vi "Finish.vi"   [LabVIEW 2020]
doc: "This VIcloses device references, sends final commands to the network tables and the joysticks, and terminates all command and control loops."
uses:
  GlobalDrivebase.vi
  GlobalDriverStationCommands.vi
  <vilib>/Rock Robotics/WPI/Utilities/WPI_GetSetVariantRefNum.vi
  GlobalMiscellaneous.vi
  GlobalActuators.vi
types:
  T1 = typedef "WPI_JoystickDevRef.ctl" = cluster{"Device":T2}
  T2 = typedef "WPI_JoystickDeviceEnum.ctl" = enum16{"USB 0", "USB 1", "USB 2", "USB 3", "USB 4", "USB 5"}
  T3 = typedef "WPI_PWMDeviceRef.ctl" = cluster{"DeviceStatus":errorcluster, "PWM Channel":T4}
  T4 = typedef "FPGA_DIOPWMChannel.ctl" = enum8{"PWM 0", "PWM 1", "PWM 2", "PWM 3", "PWM 4", "PWM 5", "PWM 6", "PWM 7", "PWM 8", "PWM 9", "PWM MXP 0", "PWM MXP 1", "PWM MXP 2", "PWM MXP 3", "PWM MXP 4", "PWM MXP 5", "PWM MXP 6", "PWM MXP 7", "PWM MXP 8", "PWM MXP 9", "Invalid"}
  T5 = typedef "WPI_MotorControlDeviceRef.ctl" = cluster{"DeviceStatus":errorcluster, "Type":T6, "PWM":cluster{"PWM Channel":T4, "DeadBand":T7}, "CAN":cluster{"Device Number":u8, "SetOutput VI Ref":variant, "GetOutput VI Ref":variant, "Enable VI Ref":variant, "Disable VI Ref":variant, "Data":variant}, "Invert":bool, "DIO PWM":cluster{"PWM \"Enable\" Channel":T4, "DIOChannel":T8, "PWM Rate":dbl}}
  T6 = typedef "WPI_MotorControlType.ctl" = enum16{"PWM", "CAN", "DIO PWM"}
  T7 = typedef "WPI_PWMDeadband.ctl" = cluster{"Name":string, "maxPositivePwm":i32, "minPositivePwm":i32, "centerPwm":i32, "maxNegativePwm":i32, "minNegativePwm":i32, "angularRange":u16}
  T8 = typedef "FPGA_DIOChannel.ctl" = enum8{"DIO 0", "DIO 1", "DIO 2", "DIO 3", "DIO 4", "DIO 5", "DIO 6", "DIO 7", "DIO 8", "DIO 9", "DIO MXP 0", "DIO MXP 1", "DIO MXP 2", "DIO MXP 3", "DIO MXP 4", "DIO MXP 5", "DIO MXP 6", "DIO MXP 7", "DIO MXP 8", "DIO MXP 9", "DIO MXP 10", "DIO MXP 11", "DIO MXP 12", "DIO MXP 13", "DIO MXP 14", "DIO MXP 15", "SPI Port CS1", "SPI Port CS2", "SPI Port CS3", "SPI Port MISO", "SPI Port MOSI", "Invalid"}
  T9 = typedef "WPI_SolenoidDevRef.ctl" = cluster{"DevStatus":errorcluster, "Pneumatics Control Module":u8, "Forward Solenoid Channel":T10, "Reverse Solenoid Channel":T10}
  T10 = typedef "WPI_SolenoidChannel.ctl" = enum8{"Solenoid 0", "Solenoid 1", "Solenoid 2", "Solenoid 3", "Solenoid 4", "Solenoid 5", "Solenoid 6", "Solenoid 7", "Solenoid 8", "Solenoid 9", "Solenoid 10", "Solenoid 11", "Solenoid 12", "Solenoid 13", "Solenoid 14", "Solenoid 15", "Invalid"}
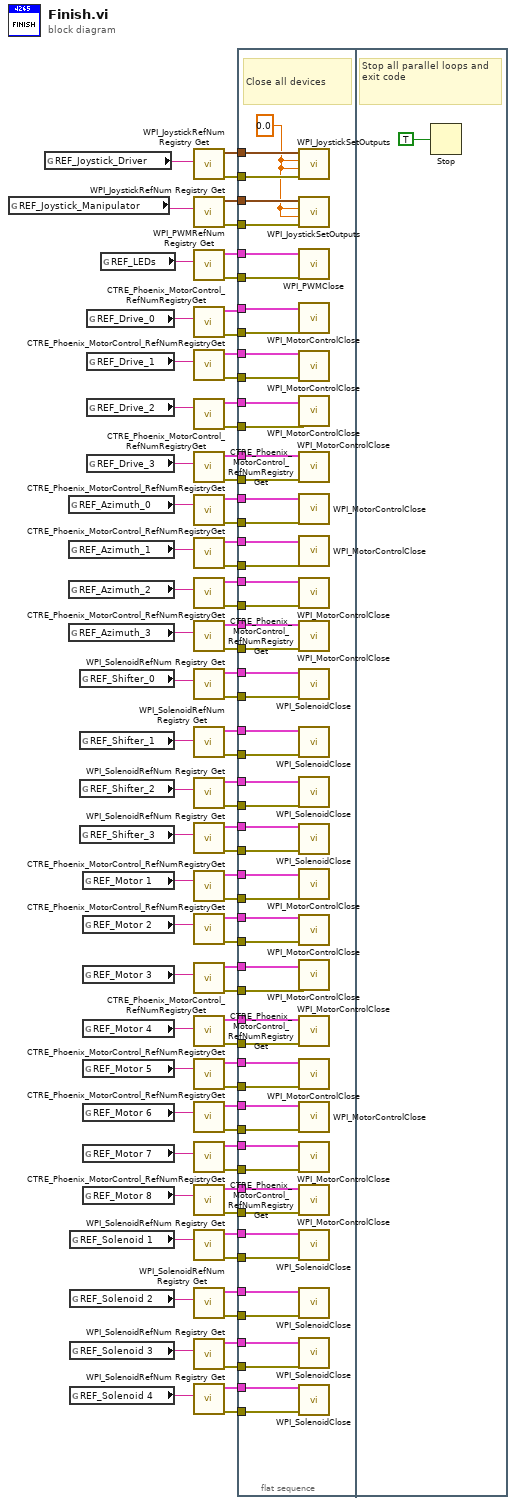
[diagram p0: block diagram]
diagram:
  n1 = global read "GlobalDriverStationCommands.vi" "REF_Joystick_Manipulator"() -> (w40:string)
  n2 = global read "GlobalDriverStationCommands.vi" "REF_Joystick_Driver"() -> (w41:string)
  n3 = global read "GlobalDrivebase.vi" "REF_Azimuth_0"() -> (w53:string)
  n4 = global read "GlobalDrivebase.vi" "REF_Azimuth_1"() -> (w52:string)
  n5 = global read "GlobalDrivebase.vi" "REF_Azimuth_2"() -> (w51:string)
  n6 = global read "GlobalDrivebase.vi" "REF_Azimuth_3"() -> (w50:string)
  n7 = global read "GlobalActuators.vi" "REF_Solenoid 1"() -> (w9:string)
  n8 = global read "GlobalActuators.vi" "REF_Solenoid 2"() -> (w10:string)
  n9 = global read "GlobalActuators.vi" "REF_Solenoid 3"() -> (w11:string)
  n10 = global read "GlobalActuators.vi" "REF_Solenoid 4"() -> (w12:string)
  n11 = global read "GlobalDrivebase.vi" "REF_Shifter_0"() -> (w45:string)
  n12 = global read "GlobalDrivebase.vi" "REF_Shifter_1"() -> (w44:string)
  n13 = global read "GlobalDrivebase.vi" "REF_Shifter_2"() -> (w43:string)
  n14 = global read "GlobalDrivebase.vi" "REF_Shifter_3"() -> (w42:string)
  n15 = global read "GlobalActuators.vi" "REF_Motor 1"() -> (w1:string)
  n16 = global read "GlobalActuators.vi" "REF_Motor 2"() -> (w2:string)
  n17 = global read "GlobalActuators.vi" "REF_Motor 3"() -> (w3:string)
  n18 = global read "GlobalActuators.vi" "REF_Motor 4"() -> (w4:string)
  n19 = global read "GlobalActuators.vi" "REF_Motor 5"() -> (w5:string)
  n20 = global read "GlobalActuators.vi" "REF_Motor 6"() -> (w6:string)
  n21 = global read "GlobalActuators.vi" "REF_Motor 7"() -> (w7:string)
  n22 = global read "GlobalActuators.vi" "REF_Motor 8"() -> (w8:string)
  n23 = global read "GlobalDrivebase.vi" "REF_Drive_0"() -> (w49:string)
  n24 = global read "GlobalDrivebase.vi" "REF_Drive_1"() -> (w48:string)
  n25 = global read "GlobalDrivebase.vi" "REF_Drive_2"() -> (w47:string)
  n26 = global read "GlobalDrivebase.vi" "REF_Drive_3"() -> (w46:string)
  n27 = global read "GlobalMiscellaneous.vi" "REF_LEDs"() -> (w37:string)
  n28 = call <vilib>:"WPI_JoystickRefNum Registry Get.vi"("refnum name"=w41) -> ("error out"=w80:errorcluster, "JoystickDevRef"=w81:T1)  [unwired: 9 in]
  n29 = call <vilib>:"WPI_JoystickRefNum Registry Get.vi"("refnum name"=w40) -> ("error out"=w78:errorcluster, "JoystickDevRef"=w79:T1)  [unwired: 9 in]
  n30 = call <vilib>:"WPI_PWMRefNum Registry Get.vi"("refnum name"=w37) -> ("error out"=w38:errorcluster, "PWMDeviceRef"=w39:T3)  [unwired: 9 in]
  n31 = call <vilib>:"CTRE_Phoenix_MotorControl_RefNumRegistryGet.vi"("refnum name"=w49) -> ("error out"=w72:errorcluster, "PhoenixMotorControlDevRef"=w73:T5)  [unwired: 9 in]
  n32 = call <vilib>:"CTRE_Phoenix_MotorControl_RefNumRegistryGet.vi"("refnum name"=w48) -> ("error out"=w68:errorcluster, "PhoenixMotorControlDevRef"=w71:T5)  [unwired: 9 in]
  n33 = call <vilib>:"CTRE_Phoenix_MotorControl_RefNumRegistryGet.vi"("refnum name"=w47) -> ("error out"=w69:errorcluster, "PhoenixMotorControlDevRef"=w70:T5)  [unwired: 9 in]
  n34 = call <vilib>:"CTRE_Phoenix_MotorControl_RefNumRegistryGet.vi"("refnum name"=w46) -> ("error out"=w76:errorcluster, "PhoenixMotorControlDevRef"=w77:T5)  [unwired: 9 in]
  n35 = call <vilib>:"CTRE_Phoenix_MotorControl_RefNumRegistryGet.vi"("refnum name"=w53) -> ("error out"=w63:errorcluster, "PhoenixMotorControlDevRef"=w67:T5)  [unwired: 9 in]
  n36 = call <vilib>:"CTRE_Phoenix_MotorControl_RefNumRegistryGet.vi"("refnum name"=w52) -> ("error out"=w62:errorcluster, "PhoenixMotorControlDevRef"=w66:T5)  [unwired: 9 in]
  n37 = call <vilib>:"CTRE_Phoenix_MotorControl_RefNumRegistryGet.vi"("refnum name"=w51) -> ("error out"=w61:errorcluster, "PhoenixMotorControlDevRef"=w65:T5)  [unwired: 9 in]
  n38 = call <vilib>:"CTRE_Phoenix_MotorControl_RefNumRegistryGet.vi"("refnum name"=w50) -> ("error out"=w60:errorcluster, "PhoenixMotorControlDevRef"=w64:T5)  [unwired: 9 in]
  n39 = call <vilib>:"WPI_SolenoidRefNum Registry Get.vi"("refnum name"=w45) -> ("error out"=w58:errorcluster, "SolenoidDevRef"=w59:T9)  [unwired: 9 in]
  n40 = call <vilib>:"WPI_SolenoidRefNum Registry Get.vi"("refnum name"=w44) -> ("error out"=w56:errorcluster, "SolenoidDevRef"=w57:T9)  [unwired: 9 in]
  n41 = call <vilib>:"WPI_SolenoidRefNum Registry Get.vi"("refnum name"=w43) -> ("error out"=w54:errorcluster, "SolenoidDevRef"=w55:T9)  [unwired: 9 in]
  n42 = call <vilib>:"WPI_SolenoidRefNum Registry Get.vi"("refnum name"=w42) -> ("error out"=w74:errorcluster, "SolenoidDevRef"=w75:T9)  [unwired: 9 in]
  n43 = call <vilib>:"CTRE_Phoenix_MotorControl_RefNumRegistryGet.vi"("refnum name"=w1) -> ("error out"=w24:errorcluster, "PhoenixMotorControlDevRef"=w23:T5)  [unwired: 9 in]
  n44 = call <vilib>:"CTRE_Phoenix_MotorControl_RefNumRegistryGet.vi"("refnum name"=w2) -> ("error out"=w28:errorcluster, "PhoenixMotorControlDevRef"=w25:T5)  [unwired: 9 in]
  n45 = call <vilib>:"CTRE_Phoenix_MotorControl_RefNumRegistryGet.vi"("refnum name"=w3) -> ("error out"=w27:errorcluster, "PhoenixMotorControlDevRef"=w26:T5)  [unwired: 9 in]
  n46 = call <vilib>:"CTRE_Phoenix_MotorControl_RefNumRegistryGet.vi"("refnum name"=w4) -> ("error out"=w22:errorcluster, "PhoenixMotorControlDevRef"=w21:T5)  [unwired: 9 in]
  n47 = call <vilib>:"CTRE_Phoenix_MotorControl_RefNumRegistryGet.vi"("refnum name"=w5) -> ("error out"=w33:errorcluster, "PhoenixMotorControlDevRef"=w29:T5)  [unwired: 9 in]
  n48 = call <vilib>:"CTRE_Phoenix_MotorControl_RefNumRegistryGet.vi"("refnum name"=w6) -> ("error out"=w34:errorcluster, "PhoenixMotorControlDevRef"=w30:T5)  [unwired: 9 in]
  n49 = call <vilib>:"CTRE_Phoenix_MotorControl_RefNumRegistryGet.vi"("refnum name"=w7) -> ("error out"=w35:errorcluster, "PhoenixMotorControlDevRef"=w31:T5)  [unwired: 9 in]
  n50 = call <vilib>:"CTRE_Phoenix_MotorControl_RefNumRegistryGet.vi"("refnum name"=w8) -> ("error out"=w36:errorcluster, "PhoenixMotorControlDevRef"=w32:T5)  [unwired: 9 in]
  n51 = call <vilib>:"WPI_SolenoidRefNum Registry Get.vi"("refnum name"=w9) -> ("error out"=w16:errorcluster, "SolenoidDevRef"=w15:T9)  [unwired: 9 in]
  n52 = call <vilib>:"WPI_SolenoidRefNum Registry Get.vi"("refnum name"=w10) -> ("error out"=w18:errorcluster, "SolenoidDevRef"=w17:T9)  [unwired: 9 in]
  n53 = call <vilib>:"WPI_SolenoidRefNum Registry Get.vi"("refnum name"=w11) -> ("error out"=w20:errorcluster, "SolenoidDevRef"=w19:T9)  [unwired: 9 in]
  n54 = call <vilib>:"WPI_SolenoidRefNum Registry Get.vi"("refnum name"=w12) -> ("error out"=w14:errorcluster, "SolenoidDevRef"=w13:T9)  [unwired: 9 in]
  n55 = flat-sequence {
    tunnel: w73 -> [w136]
    tunnel: w71 -> [w135]
    tunnel: w72 -> [w134]
    tunnel: w81 -> [w133]
    tunnel: w80 -> [w132]
    tunnel: w79 -> [w131]
    tunnel: w78 -> [w130]
    tunnel: w77 -> [w128]
    tunnel: w76 -> [w127]
    tunnel: w75 -> [w126]
    tunnel: w74 -> [w125]
    tunnel: w70 -> [w124]
    tunnel: w69 -> [w123]
    tunnel: w68 -> [w122]
    tunnel: w67 -> [w121]
    tunnel: w66 -> [w120]
    tunnel: w65 -> [w119]
    tunnel: w64 -> [w118]
    tunnel: w63 -> [w117]
    tunnel: w62 -> [w116]
    tunnel: w61 -> [w115]
    tunnel: w60 -> [w114]
    tunnel: w59 -> [w113]
    tunnel: w58 -> [w112]
    tunnel: w57 -> [w111]
    tunnel: w56 -> [w110]
    tunnel: w55 -> [w109]
    tunnel: w54 -> [w108]
    tunnel: w39 -> [w107]
    tunnel: w38 -> [w106]
    tunnel: w23 -> [w90]
    tunnel: w25 -> [w91]
    tunnel: w24 -> [w92]
    tunnel: w21 -> [w93]
    tunnel: w22 -> [w94]
    tunnel: w26 -> [w95]
    tunnel: w27 -> [w96]
    tunnel: w28 -> [w97]
    tunnel: w29 -> [w98]
    tunnel: w30 -> [w99]
    tunnel: w31 -> [w100]
    tunnel: w32 -> [w101]
    tunnel: w33 -> [w102]
    tunnel: w34 -> [w103]
    tunnel: w35 -> [w104]
    tunnel: w36 -> [w105]
    tunnel: w13 -> [w82]
    tunnel: w14 -> [w83]
    tunnel: w15 -> [w84]
    tunnel: w16 -> [w85]
    tunnel: w17 -> [w86]
    tunnel: w18 -> [w87]
    tunnel: w19 -> [w88]
    tunnel: w20 -> [w89]
    frame #0 {
      w129 = sgl 0.0 ("Left Rumble")
      # "Close all devices"
      n56 = call <vilib>:"WPI_JoystickSetOutputs.vi"("error in (no error)"=w132, "Right Rumble"=w129, "Left Rumble"=w129, "JoystickDevRef"=w133) -> ()  [unwired: 6 in, 2 out]
      n57 = call <vilib>:"WPI_JoystickSetOutputs.vi"("error in (no error)"=w130, "Right Rumble"=w129, "Left Rumble"=w129, "JoystickDevRef"=w131) -> ()  [unwired: 6 in, 2 out]
      n58 = call <vilib>:"WPI_PWMClose.vi"("error in (no error)"=w106, "PWMDeviceRef"=w107) -> ()  [unwired: 9 in, 1 out]
      n59 = call <vilib>:"WPI_MotorControlClose.vi"("error in"=w134, "MotorControlDevRef"=w136) -> ()  [unwired: 9 in, 1 out]
      n60 = call <vilib>:"WPI_MotorControlClose.vi"("error in"=w122, "MotorControlDevRef"=w135) -> ()  [unwired: 9 in, 1 out]
      n61 = call <vilib>:"WPI_MotorControlClose.vi"("error in"=w123, "MotorControlDevRef"=w124) -> ()  [unwired: 9 in, 1 out]
      n62 = call <vilib>:"WPI_MotorControlClose.vi"("error in"=w127, "MotorControlDevRef"=w128) -> ()  [unwired: 9 in, 1 out]
      n63 = call <vilib>:"WPI_MotorControlClose.vi"("error in"=w117, "MotorControlDevRef"=w121) -> ()  [unwired: 9 in, 1 out]
      n64 = call <vilib>:"WPI_MotorControlClose.vi"("error in"=w116, "MotorControlDevRef"=w120) -> ()  [unwired: 9 in, 1 out]
      n65 = call <vilib>:"WPI_MotorControlClose.vi"("error in"=w115, "MotorControlDevRef"=w119) -> ()  [unwired: 9 in, 1 out]
      n66 = call <vilib>:"WPI_MotorControlClose.vi"("error in"=w114, "MotorControlDevRef"=w118) -> ()  [unwired: 9 in, 1 out]
      n67 = call <vilib>:"WPI_SolenoidClose.vi"("error in (no error)"=w112, "SolenoidDevRef"=w113) -> ()  [unwired: 9 in, 1 out]
      n68 = call <vilib>:"WPI_SolenoidClose.vi"("error in (no error)"=w110, "SolenoidDevRef"=w111) -> ()  [unwired: 9 in, 1 out]
      n69 = call <vilib>:"WPI_SolenoidClose.vi"("error in (no error)"=w108, "SolenoidDevRef"=w109) -> ()  [unwired: 9 in, 1 out]
      n70 = call <vilib>:"WPI_SolenoidClose.vi"("error in (no error)"=w125, "SolenoidDevRef"=w126) -> ()  [unwired: 9 in, 1 out]
      n71 = call <vilib>:"WPI_MotorControlClose.vi"("error in"=w92, "MotorControlDevRef"=w90) -> ()  [unwired: 9 in, 1 out]
      n72 = call <vilib>:"WPI_MotorControlClose.vi"("error in"=w97, "MotorControlDevRef"=w91) -> ()  [unwired: 9 in, 1 out]
      n73 = call <vilib>:"WPI_MotorControlClose.vi"("error in"=w96, "MotorControlDevRef"=w95) -> ()  [unwired: 9 in, 1 out]
      n74 = call <vilib>:"WPI_MotorControlClose.vi"("error in"=w94, "MotorControlDevRef"=w93) -> ()  [unwired: 9 in, 1 out]
      n75 = call <vilib>:"WPI_MotorControlClose.vi"("error in"=w102, "MotorControlDevRef"=w98) -> ()  [unwired: 9 in, 1 out]
      n76 = call <vilib>:"WPI_MotorControlClose.vi"("error in"=w103, "MotorControlDevRef"=w99) -> ()  [unwired: 9 in, 1 out]
      n77 = call <vilib>:"WPI_MotorControlClose.vi"("error in"=w104, "MotorControlDevRef"=w100) -> ()  [unwired: 9 in, 1 out]
      n78 = call <vilib>:"WPI_MotorControlClose.vi"("error in"=w105, "MotorControlDevRef"=w101) -> ()  [unwired: 9 in, 1 out]
      n79 = call <vilib>:"WPI_SolenoidClose.vi"("error in (no error)"=w85, "SolenoidDevRef"=w84) -> ()  [unwired: 9 in, 1 out]
      n80 = call <vilib>:"WPI_SolenoidClose.vi"("error in (no error)"=w87, "SolenoidDevRef"=w86) -> ()  [unwired: 9 in, 1 out]
      n81 = call <vilib>:"WPI_SolenoidClose.vi"("error in (no error)"=w89, "SolenoidDevRef"=w88) -> ()  [unwired: 9 in, 1 out]
      n82 = call <vilib>:"WPI_SolenoidClose.vi"("error in (no error)"=w83, "SolenoidDevRef"=w82) -> ()  [unwired: 9 in, 1 out]
    }
    frame #1 {
      # "Stop all parallel loops and exit code"
      n83 = Stop(stop? (T)=TRUE ("Quit")) -> ()
    }
  }
